vi "Flush.vi"(8 "error in (no error)":errorcluster) -> (0 "error out":errorcluster, 2 "No. Of Remaining Elements":i32, 3 "Remaining Elements":T1[](array[typedef]))   [LabVIEW 2022 SP3]
doc: "Flushes (dequeues) all the elements from the queue. The queue is empty immediately after this VI executes."
uses:
  Message.ctl
  Command.ctl
panel:
  # "Development\ncontrols/indicators useful for development and testing, but which are not outputs of the VI"
  # "Input\nInputs to the VI"
  # "Output\nOutputs of the VI"
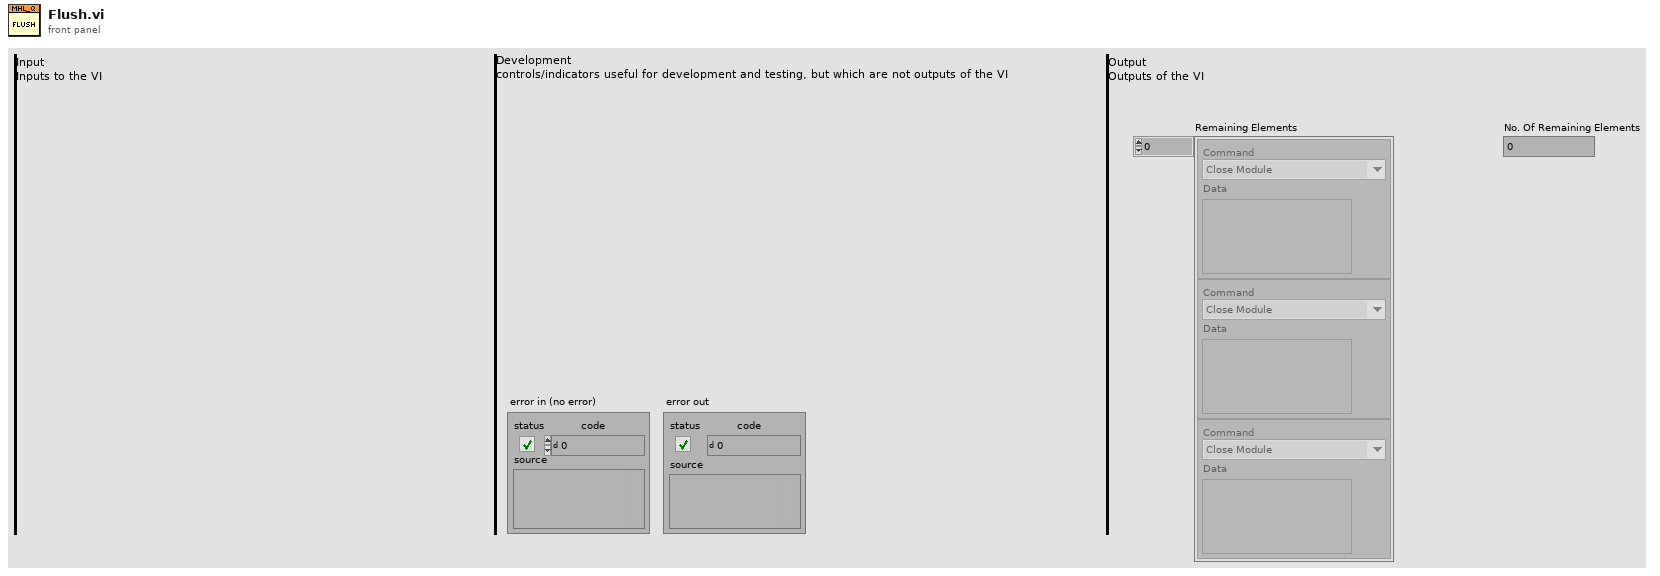
[diagram p1: front panel]
types:
  T1 = typedef "Message.ctl" = cluster{"Command":T2, "Data":variant}
  T2 = typedef "Command.ctl" = enum16{"Init Module", "Close Module", "Local Error Handler", "Command 1 (replace me)", "Command 2 (replace me)", "Command 3 (replace me)"}
  T3 = typedef "AsyncModuleTemplate.lvlib/MhlQueue.lvlib/Message.ctl" = cluster{"Command":T4, "Data":variant}
  T4 = typedef "AsyncModuleTemplate.lvlib/MhlQueue.lvlib/Command.ctl" = enum16{"Init Module", "Close Module", "Local Error Handler", "Command 1 (replace me)", "Command 2 (replace me)", "Command 3 (replace me)"}
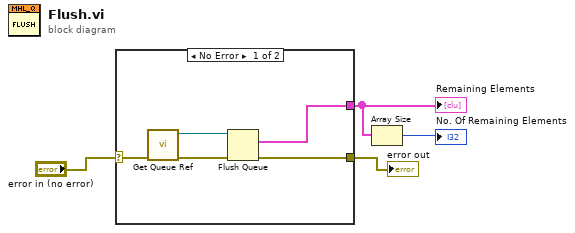
[diagram p0: block diagram]
diagram:
  n1 = case shown="No Error" "error in (no error)" {
    selector: "error in (no error)" -> [w9 w10]
    tunnel: [w8 w10] -> w3
    tunnel: [w5 _] -> w2
    frame No Error {
      n2 = call "Get Queue Ref.vi"("error in (no error)"=w9) -> ("error out"=w6:errorcluster, "Queue Ref"=w7:refnum<queue>)  [unwired: 9 in]
      n3 = Flush Queue(queue=w7, error in (no error)=w6) -> (remaining elements=w5:T3[], error out=w8:errorcluster)  [unwired: 1 out]
    }
    frame Error {
    }
  }
  "error out" <- w3
  "Remaining Elements" <- w2
  n4 = Array Size(array=w2) -> (size(s)=→"No. Of Remaining Elements":i32)
